vi "_004.vi"() -> ()   [LabVIEW 2024]
panel:
  out "Not":bool
  out "Xor":bool
  out "Nor":bool
  out "Or":bool
  out "Nandnd":bool
  in  "B":bool
  out "And":bool
  in  "A":bool
  # "Symbols & Truth Table for LOGIC GATES :"
  # "A  B   And\n0  0  -> 0\n0  1   -> 0\n1   0  -> 0\n1   1   ->  1"
  # "A  B    Nand\n0  0  -> 1\n0  1   -> 1\n1   0  -> 1\n1   1   -> 0"
  # "A  B    Or\n0  0  -> 0\n0  1   ->  1\n1   0  ->  1\n1   1   ->  1"
  # "A  B    Nor\n0  0  -> 1\n0  1   -> 0\n1   0  -> 0\n1   1   -> 0"
  # "A  B    Xor\n0  0  -> 0\n0  1   ->  1\n1   0  ->  1\n1   1   -> 0"
  # "A    Not   \n0  -> 1\n1   -> 0"
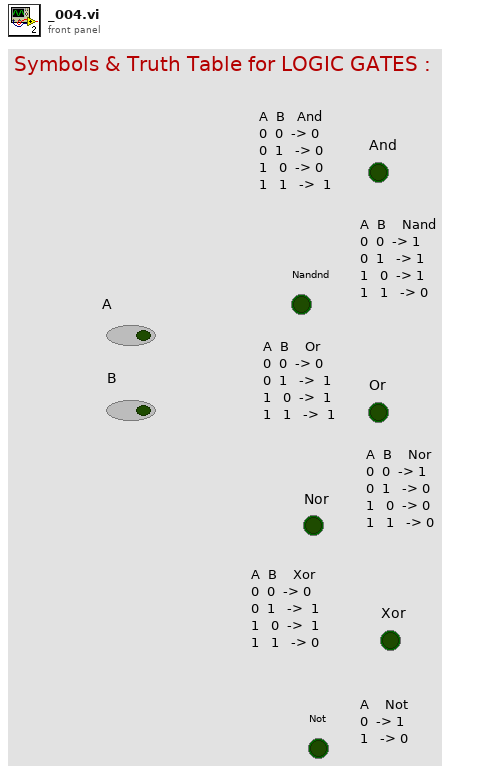
[diagram p1: front panel]
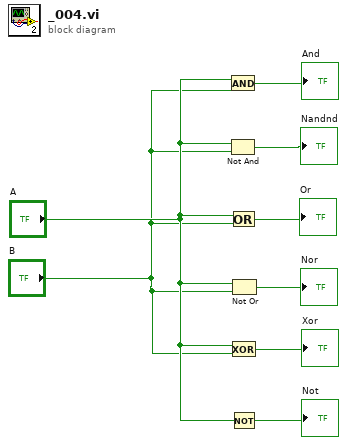
[diagram p0: block diagram]
diagram:
  n1 = And(x="A", y="B") -> (x .and. y?=→"And":bool)
  n2 = Not And(1:"B", 2:"A") -> (0:→"Nandnd":bool)
  n3 = Or(x="A", y="B") -> (x .or. y?=→"Or":bool)
  n4 = Not Or(1:"B", 2:"A") -> (0:→"Nor":bool)
  n5 = Exclusive Or(1:"B", 2:"A") -> (0:→"Xor":bool)
  n6 = Not(x="A") -> (.not. x?=→"Not":bool)
